vi "Phasor Compute Calibration Map Size.vi"(11 "Center Coordinates":cluster{"X":i32, "Y":i32}[](array[cluster])) -> (1 "Map Resolution Y":i32, 3 "Map Resolution X":i32)   [LabVIEW 2021, in "Phasor.lvlib"]
uses:
  Phasor.lvlib
  d4c31e8f-ea48-4089-b4b5-7cf5844691c2.vi
  5183907f-9671-479a-a59f-9a137911e8cd.vi
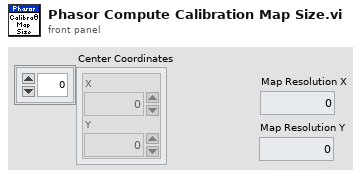
[diagram p1: front panel]
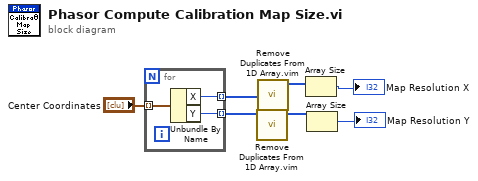
[diagram p0: block diagram]
diagram:
  n1 = for {
    tunnel: "Center Coordinates" -> [w10] mode=indexing
    tunnel: [w9] -> w6 mode=indexing
    tunnel: [w8] -> w5 mode=indexing
    n2 = Unbundle By Name(w10) -> ("X"=w9:i32, "Y"=w8:i32)
  }
  n3 = call "Remove Duplicates From 1D Array.vim"("array"=w5) -> ("array with duplicates removed"=w3:i32[])  [unwired: 10 in]
  n4 = call "Remove Duplicates From 1D Array.vim"("array"=w6) -> ("array with duplicates removed"=w4:i32[])  [unwired: 10 in]
  n5 = Array Size(array=w4) -> (size(s)=→"Map Resolution X":i32)
  n6 = Array Size(array=w3) -> (size(s)=→"Map Resolution Y":i32)
